vi "Stop Dependency.vi"(6 "Destroy ref? (T)":bool=TRUE, 8 "error in (no error)":errorcluster, 9 "Name (ignored if reference valid)":string, 10 "Dependency Reference":refnum<class "SMO.lvclass">, 11 "SMO in":refnum<class "SMO.lvclass">) -> (0 "error out":errorcluster, 2 "Dependency Reference out":refnum<class "SMO.lvclass">, 3 "SMO out":refnum<class "SMO.lvclass">)   [LabVIEW 2013, in "SMO.lvclass"]
uses:
  SMO.lvclass
  Support/Attribute.Owner/Attribute.Owner.lvclass
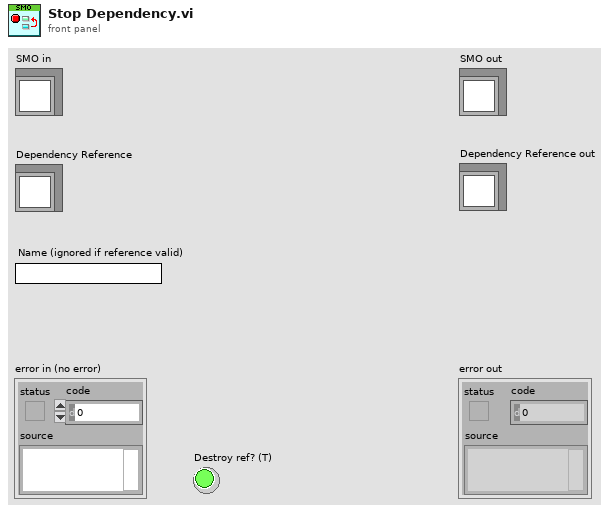
[diagram p1: front panel]
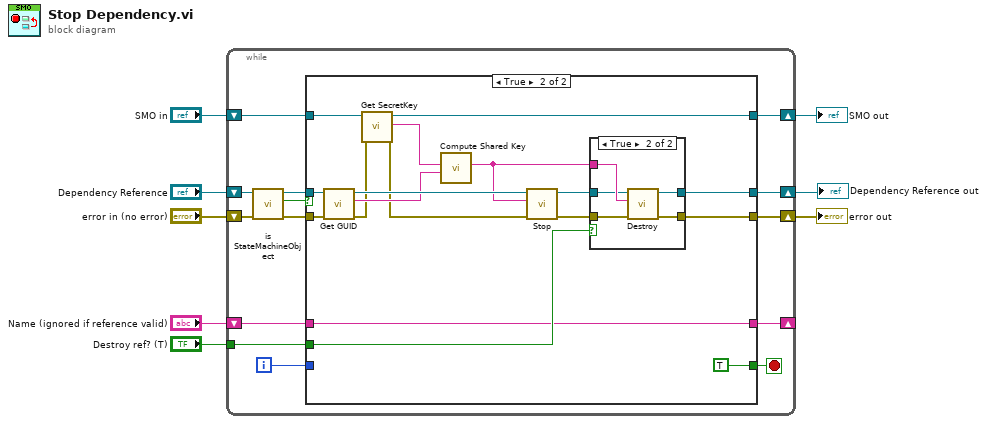
[diagram p0: block diagram]
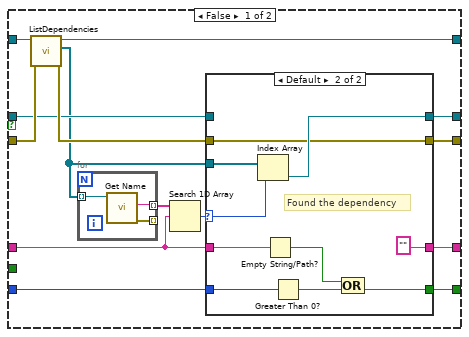
[diagram p2: hidden frame]
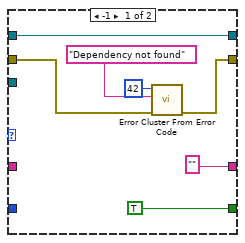
[diagram p3: hidden frame]
diagram:
  n1 = while {
    tunnel: "Destroy ref? (T)" -> [w13]
    shift-right: [w12] -> w1
    shift-left: "Dependency Reference" -> [w19]
    shift-right: [w22] -> w8
    shift-left: "error in (no error)" -> [w18]
    shift-right: [w20] -> w6
    shift-left: "SMO in" -> [w21]
    shift-right: [w9] -> _
    shift-left: "Name (ignored if reference valid)" -> [w14]
    i -> [w10]
    stop <- w11 stop-if-true
    n2 = call "is StateMachineObject.vi"("error in (no error)"=w18, "SMO"=w19) -> ("error out"=w17:errorcluster, "is SMO?"=w16:bool, "SMO out"=w15:refnum<class "SMO.lvclass">)  [unwired: 7 in]
    n3 = case shown="True" w16 {
      tunnel: [w31 w60] -> w22
      tunnel: w21 -> [w36 w73]
      tunnel: [w35 w70] -> w20
      tunnel: w17 -> [w34 w67]
      tunnel: w15 -> [w28 w72]
      tunnel: w14 -> [w23 w57]
      tunnel: w13 -> [_ w61]
      tunnel: [w29 w59] -> w12
      tunnel: [w27 TRUE] -> w11
      tunnel: w10 -> [w25 _]
      tunnel: [w24 w57] -> w9
      frame False {
        n4 = call "ListDependencies.vi"("error in (no error)"=w34, "SMO in"=w36) -> ("error out"=w30:errorcluster, "[Dependencies]"=w26:refnum<class "SMO.lvclass">[], "SMO out"=w35:refnum<class "SMO.lvclass">)  [unwired: 6 in, 1 out]
        n5 = for {
          tunnel: w26 -> [w56] mode=indexing
          tunnel: [w55] -> w33 mode=indexing
          tunnel: [w54] -> _ mode=indexing
          n6 = call "Get Name.vi"("SMO"=w56) -> ("error out"=w54:errorcluster, "Name"=w55:string)  [unwired: 8 in, 1 out]
        }
        n7 = Search 1D Array(1D array=w33, element=w23) -> (index of element=w32:i32)  [unwired: 1 in]
        n8 = case shown="Default" w32 {
          selector: w32 -> [_ w50]
          tunnel: [w40 w51] -> w31
          tunnel: w30 -> [w41 w51]
          tunnel: [w43 w52] -> w29
          tunnel: w28 -> [w43 _]
          tunnel: [TRUE w44] -> w27
          tunnel: w26 -> [_ w53]
          tunnel: w25 -> [_ w49]
          tunnel: ["" ("error message (\"\")") "" ("error message (\"\")")] -> w24
          tunnel: w23 -> [_ w47]
          frame -1 {
            n9 = call <vilib>:"Error Cluster From Error Code.vi"("error in (no error)"=w41, "error message (\"\")"="Dependency not found" ("error message (\"\")"), "error code (0)"=42) -> ("error out"=w40:errorcluster)  [unwired: 6 in]
          }
          frame Default {
            # "Found the dependency"
            n10 = Index Array(array=w53, index=w50) -> (element=w52:refnum<class "SMO.lvclass">)
            n11 = Empty String/Path?(string/path=w47) -> (empty?=w46:bool)
            n12 = Greater Than 0?(x=w49) -> (x > 0?=w45:bool)
            n13 = Compound Arithmetic op=OR(w46, w45) -> (w44:bool)
          }
        }
      }
      frame True {
        n14 = call "Get GUID.vi"("error in (no error)"=w67, "SMO"=w72) -> ("error out"=w66:errorcluster, "GUID"=w68:string, "SMO out"=w71:refnum<class "SMO.lvclass">)  [unwired: 7 in]
        n15 = call "Get SecretKey.vi"("error in (no error)"=w66, "SMO"=w73) -> ("error out"=w65:errorcluster, "SecretKey"=w69:string, "SMO out"=w70:refnum<class "SMO.lvclass">)  [unwired: 7 in]
        n16 = call "Compute Shared Key.vi"("GUID"=w68, "SecretKey"=w69) -> ("Shared Key"=w62:string)  [unwired: 9 in]
        n17 = call "Stop.vi"("error in (no error)"=w65, "Shared Key"=w62, "SMO"=w71) -> ("error out"=w63:errorcluster, "SMO out"=w64:refnum<class "SMO.lvclass">)  [unwired: 7 in]
        n18 = case shown="True" w61 {
          tunnel: w64 -> [w75 w76]
          tunnel: w63 -> [w74 w79]
          tunnel: w62 -> [_ w78]
          tunnel: [w74 w77] -> w60
          tunnel: [w75 w76] -> w59
          frame False {
          }
          frame True {
            n19 = call "Destroy.vi"("error in (no error)"=w79, "Shared Key"=w78, "SMO"=w76) -> ("error out"=w77:errorcluster)  [unwired: 8 in]
          }
        }
      }
    }
  }
  "error out" <- w8
  "SMO out" <- w6
  "Dependency Reference out" <- w1
